vi "Create Polynomial from Roots of Unity.vi"() -> ()   [LabVIEW 2023]
doc: "This example shows how to create a polynomial from roots of unity."
uses:
  <vilib>/Analysis/1siggen.llb/Ramp Pattern by Samples.vi
  <vilib>/Analysis/polynomials.llb/Create Polynomial From Roots (CDB).vi
  <vilib>/Analysis/NI_AALPro.lvlib
  <vilib>/Analysis/NI_AALBase.lvlib
panel:
  out "rendered equation":picture
  in  "Stop":bool
  out "Roots Distribution":cdb[](graph)
  out "Polynomial Coefficients":dbl[](graph)
  in  "Number of Roots":i32(slide)=20 scale=1.0..25.0
  # "Overview: Demonstrates how to create a polynomial from roots with the Create Polynomial From Roots VI.\nRequirements: LabVIEW Full Development System\nInstructions:\n1. Run the VI.\n2. Change the Number of Roots, and view the change of Polynomial Coefficients.\n3. Click Stop to stop the VI."
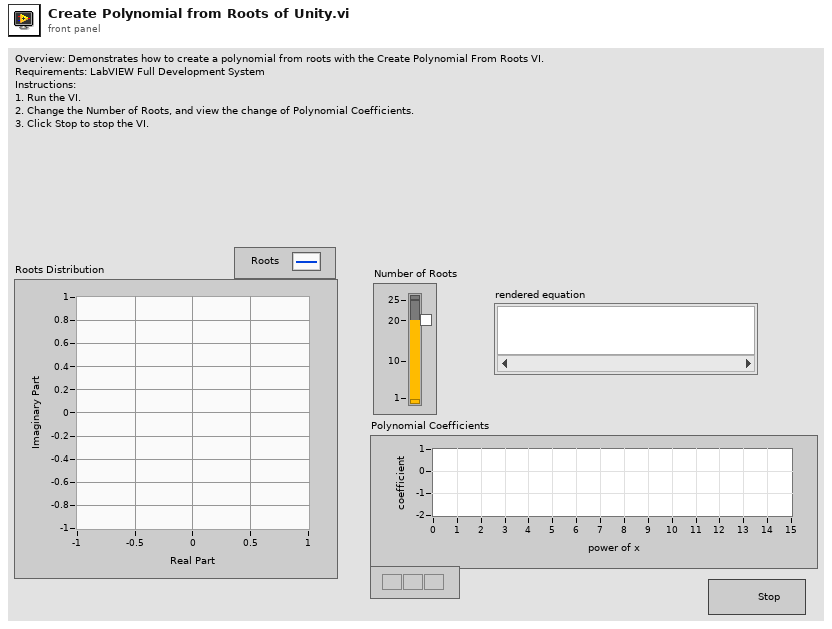
[diagram p1: front panel]
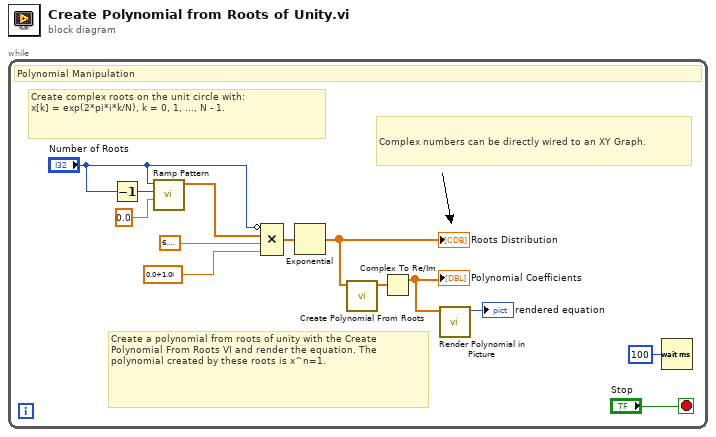
[diagram p0: block diagram]
diagram:
  n1 = while {
    stop <- "Stop" stop-if-true
    # "Complex numbers can be directly wired to an XY Graph."
    # "Create complex roots on the unit circle with:\nx[k] = exp(2*pi*i*k/N), k = 0, 1, ..., N - 1."
    # "Create a polynomial from roots of unity with the Create Polynomial From Roots VI and render the equation. The polynomial created by these roots is x^n=1."
    # "Polynomial Manipulation"
    n2 = Decrement(x="Number of Roots") -> (x-1=w12:i32)
    n3 = call-poly <vilib>:"Ramp Pattern.vi"("start"=0.0, "end"=w12, "samples"="Number of Roots") -> ("Ramp Pattern"=w9:dbl[])  [unwired: 7 in, 1 out]
    n4 = Compound Arithmetic op=MULTIPLY(invert "Number of Roots", w9, 6.283185307179586, cdb 0.0+1.0i) -> (w3:cdb[])
    n5 = Exponential(1:w3) -> (0:w5:cdb[])
    "Roots Distribution" <- w5
    n6 = call-poly <vilib>:"Create Polynomial From Roots.vi"("Roots"=w5) -> ("P(x)"=w6:cdb[])  [unwired: 9 in, 1 out]
    n7 = Complex To Re/Im(x + iy=w6) -> (x=w4:dbl[])  [unwired: 1 out]
    "Polynomial Coefficients" <- w4
    n8 = call "Render Polynomial in Picture.vi"("coefficients"=w4) -> ("rendered equation"=→"rendered equation":picture)  [unwired: 10 in]
    n9 = Wait (ms)(milliseconds to wait=u32 100) -> ()  [unwired: 1 out]
  }
